vi "stableEdge.vi"(8 "Stable Time":dbl, 11 "current":bool) -> (3 "Output":bool)   [LabVIEW 2012]
panel:
  in  "Start":bool
  out "Ref Time Stamp":timestamp
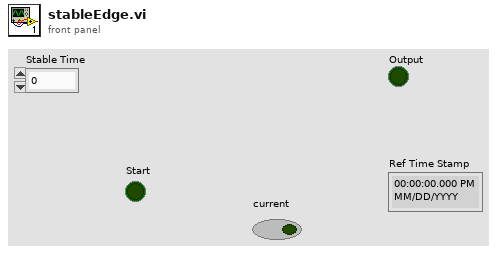
[diagram p1: front panel]
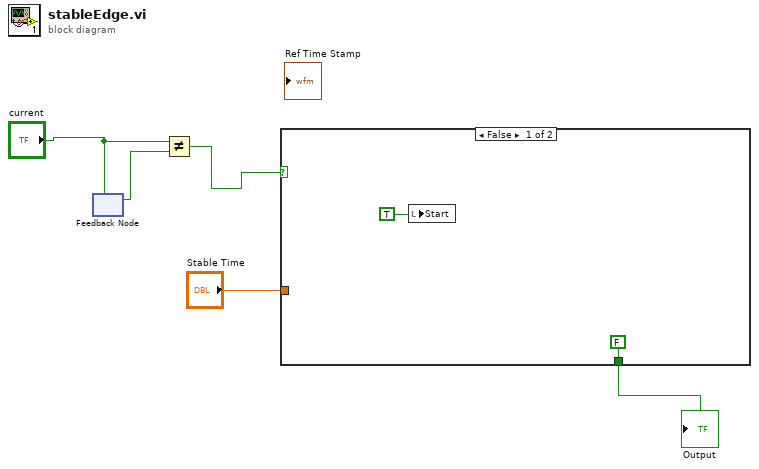
[diagram p0: block diagram]
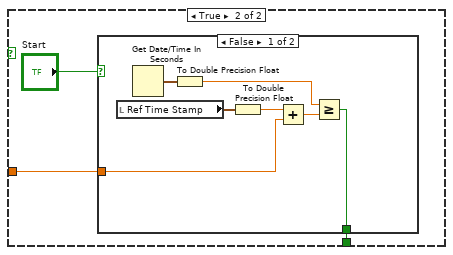
[diagram p2: hidden frame]
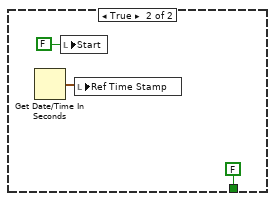
[diagram p3: hidden frame]
diagram:
  n1 = feedback #1() -> (w4:bool)  [unwired: 1 in]
  n2 = feedback-in #1("current") -> ()
  n3 = Not Equal?(x="current", y=w4) -> (x != y?=w3:bool)
  n4 = case shown="False" w3 {
    tunnel: [FALSE w10] -> w1
    tunnel: "Stable Time" -> [_ w9]
    frame False {
      n5 = local write "Start"(TRUE) -> ()
    }
    frame True {
      n6 = case shown="False" "Start" {
        tunnel: [w12 FALSE] -> w10
        tunnel: w9 -> [w11 _]
        frame False {
          n7 = local read "Ref Time Stamp"() -> (w16:timestamp)
          n8 = Get Date/Time In Seconds() -> (seconds since 1Jan1904=w17:timestamp)
          n9 = To Double Precision Float(number=w17) -> (double precision float=w13:dbl)
          n10 = To Double Precision Float(number=w16) -> (double precision float=w15:dbl)
          n11 = Add(x=w15, y=w11) -> (x+y=w14:dbl)
          n12 = Greater Or Equal?(x=w13, y=w14) -> (x >= y?=w12:bool)
        }
        frame True {
          n13 = Get Date/Time In Seconds() -> (seconds since 1Jan1904=w20:timestamp)
          n14 = local write "Start"(FALSE ("Start")) -> ()
          n15 = local write "Ref Time Stamp"(w20) -> ()
        }
      }
    }
  }
  "Output" <- w1
